vi "Comm Error Check1 (SubVI).vi"(8 "error in (no error)":errorcluster, 10 "Error Source String":string, 11 "result string":string) -> ()   [LabVIEW 2020]
doc: "Checks instrument reply message (must be wired to the \"result string\" input terminal) and looking for \"ERROR#\" string. If found displays dialog box with message string wired to the \"Error Source String\" terminal. This SubVI will block program execution if instrument replies with error message. If your application should not be interrupted do not use this SubVI."
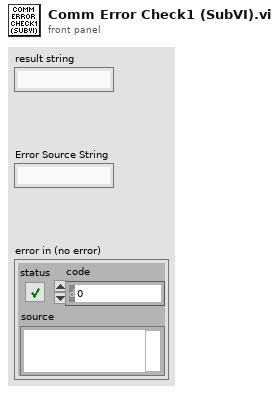
[diagram p1: front panel]
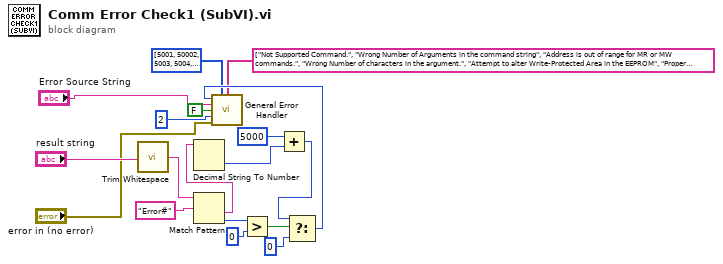
[diagram p0: block diagram]
diagram:
  n1 = call <vilib>:"Trim Whitespace.vi"("string"="result string") -> ("trimmed string"=w16:string)  [unwired: 1 in]
  n2 = Match Pattern(string=w16, regular expression="Error#") -> (after substring=w12:string, offset past match=w14:i32)  [unwired: 1 in, 2 out]
  n3 = Decimal String To Number(string=w12) -> (number=w1:i32)  [unwired: 2 in, 1 out]
  n4 = Greater?(x=w14, y=0) -> (0:w18:bool)
  n5 = Add(x=5000, y=w1) -> (x+y=w2:i32)
  n6 = Select(t=w2, s=w18, f=0) -> (s? t:f=w10:i32)
  n7 = call <vilib>:"General Error Handler.vi"("[error code] (0)"=w10, "[user-defined codes]"=i32[] [5001, 50002, 5003, 5004, 5005, 5006, 5007, 5008, 5009], "[user-defined descriptions]"=string[] ["Not Supported Command.", "Wrong Number of Arguments in the command string", "Address is out of range for MR or MW commands.", "Wrong Number of characters in the argument.", "Attempt to alter Write-Protected Area in the EEPROM", "Proper Command or Argument not found", "Wrong value of the Argument in the command string.", "Wrong value of the Argument", "Manufacturer-specific information EE access KEY (wrong key or key is disabled.", "No Description evailable for this Error code."], "[error source] (\" \")"="Error Source String", "search ni.com link visible?(T)"=FALSE, "type of dialog (OK msg:1)"=2, "error in (no error)"="error in (no error)") -> ()  [unwired: 4 in, 5 out]
